vi "FTP_CheckUpload.vi"(2 "reply string":string, 3 "file path (<NAP>)":path=path "") -> (0 "same size?":bool, 1 "On server?":bool)   [LabVIEW 2012]
panel:
  out "file elements":string[](array[string])
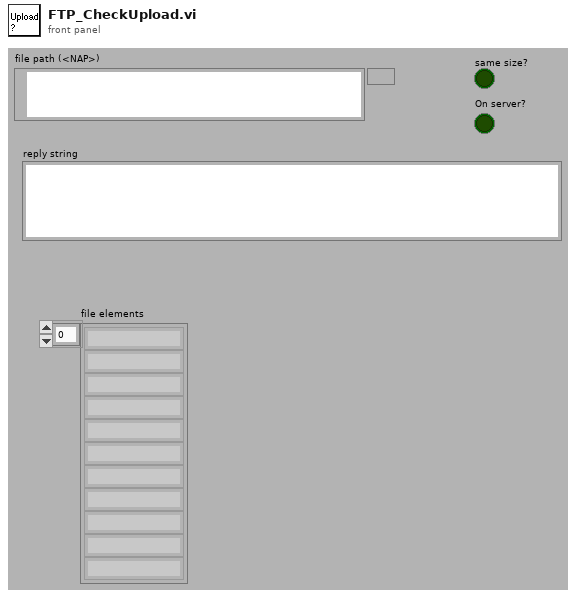
[diagram p1: front panel]
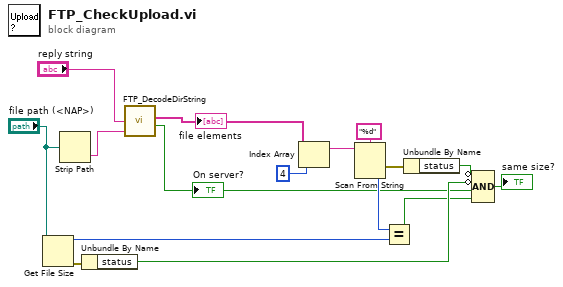
[diagram p0: block diagram]
diagram:
  n1 = Get File Size(file="file path (<NAP>)") -> (size (in bytes)=w9:i64, 0:w5:errorcluster)  [unwired: 1 in, 1 out]
  n2 = Strip Path(path="file path (<NAP>)") -> (name=w15:string)  [unwired: 1 out]
  n3 = Unbundle By Name(w5) -> ("status"=w4:bool)
  n4 = call <userlib>:"FTP_DecodeDirString.vi"("directory"="reply string", "name"=w15) -> ("file elements"=w14:string[], "On Server?"=w3:bool)  [unwired: 4 out]
  "On server?" <- w3
  "file elements" <- w14
  n5 = Index Array(array=w14, index=4) -> (element=w12:string)
  n6 = Scan From String(format string="%d", input string=w12) -> (error out=w7:errorcluster, output 1=w10:i32)  [unwired: 2 in, 3 out]
  n7 = Equal?(x=w10, y=w9) -> (x = y?=w2:bool)
  n8 = Unbundle By Name(w7) -> ("status"=w6:bool)
  n9 = Compound Arithmetic op=AND(invert w6, invert w4, w3, w2) -> (→"same size?":bool)
